vi "Frames.vi"(8 "error in (no error)":errorcluster, 11 "Node Ptr":T1 format="%.0x") -> (0 "error out":errorcluster)   [LabVIEW 2019, in "Diagnostics Addon System Explorer.lvlib"]
uses:
  Diagnostics Addon System Explorer.lvlib
  <vilib>/NI VeriStand/Custom Device API/Custom Device Item Ref.ctl
  Types/FG.Action.ctl
  Addon Shared/SubVIs/Constants.vi
  <vilib>/NI/NI VeriStand Advanced SysDef API/SysDef API/SysDef.Property.Set.vi
  <vilib>/NI/NI VeriStand Advanced SysDef API/_SubVIs/SysDef.Property.Set.U32.vi
  <vilib>/NI VeriStand/Custom Device API/NI VeriStand - Get Item Property.vi
  <vilib>/NI VeriStand/Custom Device API/Get Item Property (U32).vi
  <vilib>/NI VeriStand/Custom Device API/Custom Device API.lvlib
  Addon Shared/Diagnostics Addon Shared.lvlib
panel:
  in  "Description":string
  in  "SHDocVw.IWebBrowser":refnum<k7>(container)
  out "Frames":i32(listbox)
  out "Name":string
  in  "Header":cluster{"Section Name":string}={"Section Name"="Custom Device Item Settings"}
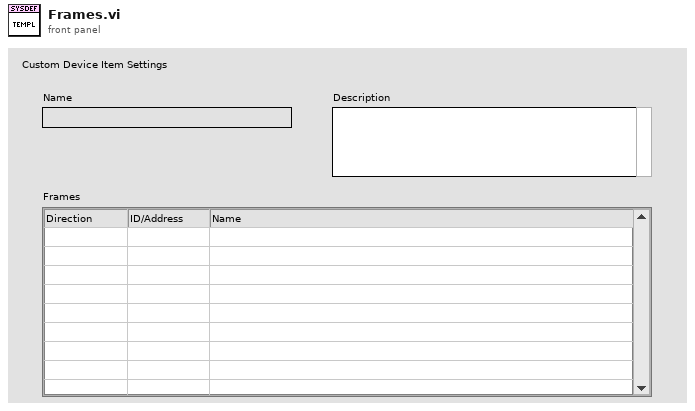
[diagram p1: front panel]
types:
  T1 = typedef "Custom Device API.lvlib/Custom Device Item Ref.ctl" = u64
  T2 = typedef "Diagnostics Addon System Explorer.lvlib/FG.Action.ctl" = enum16{"Get", "Set"}
  T3 = typedef "Custom Device API.lvlib/Custom Device Item Info.ctl" = cluster{"Name":string, "Is Channel":bool, "GUID":string, "Is Waveform":bool}
  T4 = typedef "Custom Device API.lvlib/Custom Device Commands.ctl" = enum16{"Default", "Item renamed", "Shutdown", "Dynamic button pressed"}
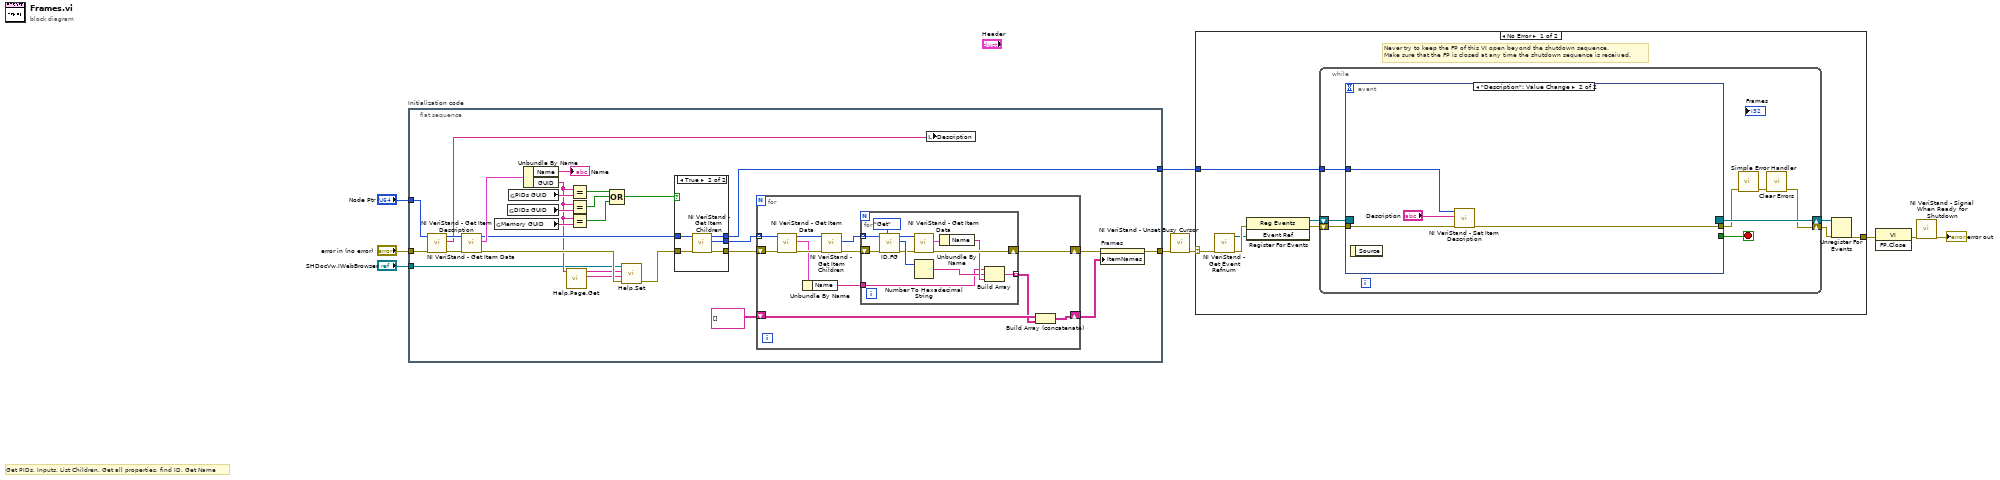
[diagram p0: block diagram]
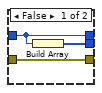
[diagram p2: hidden frame]
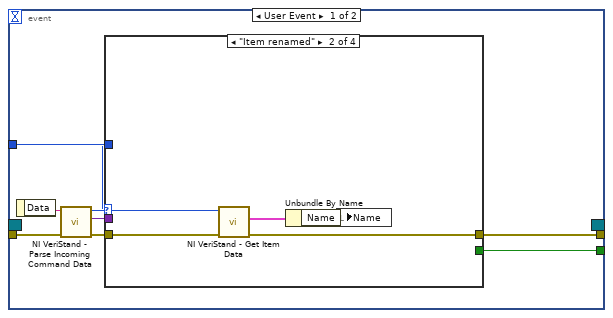
[diagram p3: hidden frame]
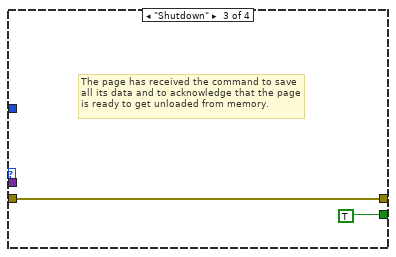
[diagram p5: hidden frame]
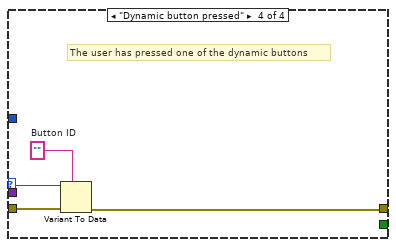
[diagram p6: hidden frame]
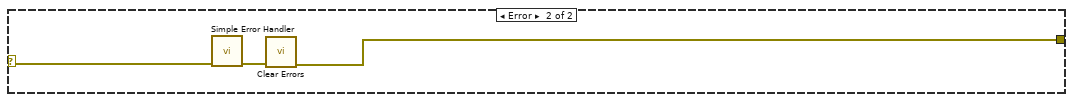
[diagram p7: hidden frame]
diagram:
  # "Get PIDs, Inputs, List Children, Get all properties, find ID, Get Name"
  n1 = flat-sequence "Initialization code" {
    tunnel: "error in (no error)" -> [w23]
    tunnel: "Node Ptr" -> [w36]
    tunnel: [w32] -> w5
    tunnel: [w29] -> w2
    tunnel: "SHDocVw.IWebBrowser" -> [w11]
    frame #0 {
      n2 = call <vilib>:"NI VeriStand - Get Item Description.vi"("error in (no error)"=w23, "Item Ref in"=w36) -> ("error out"=w35:errorcluster, "Description"=w24:string, "Item Ref out"=w37:T1)  [unwired: 7 out]
      n3 = call <vilib>:"NI VeriStand - Get Item Data.vi"("error in (no error)"=w35, "Item Ref in"=w37) -> ("error out"=w22:errorcluster, "Item Info"=w34:T3, "Item Ref out"=w31:T1)  [unwired: 7 out]
      n4 = global read "Constants.vi" "Memory GUID"() -> (w18:string)
      n5 = global read "Constants.vi" "DIDs GUID"() -> (w16:string)
      n6 = global read "Constants.vi" "PIDs GUID"() -> (w15:string)
      n7 = Unbundle By Name(w34) -> ("Name"=→"Name":string, "GUID"=w13:string)
      n8 = call "Help.Page.Get.vi"("GUID"=w13) -> ("HTML File"=w12:string, "Main CHM File"=w10:string)  [unwired: 9 in]
      n9 = Equal?(x=w13, y=w15) -> (x = y?=w20:bool)
      n10 = Equal?(x=w13, y=w16) -> (x = y?=w17:bool)
      n11 = Equal?(x=w13, y=w18) -> (x = y?=w19:bool)
      n12 = Compound Arithmetic op=OR(w20, w17, w19) -> (w14:bool)
      n13 = call "Help.Set.vi"("error in (no error)"=w22, "HTML File"=w12, "Main CHM File"=w10, "SHDocVw.IWebBrowser2"=w11) -> ("error out"=w21:errorcluster)  [unwired: 7 in]
      n14 = case shown="True" w14 {
        tunnel: w21 -> [w40 w45]
        tunnel: w31 -> [w39 w44]
        tunnel: [w40 w43] -> w30
        tunnel: [w39 w42] -> w29
        tunnel: [w38 w41] -> w28
        frame False {
          n15 = Build Array(w39) -> (w38:T1[])
        }
        frame True {
          n16 = call <vilib>:"NI VeriStand - Get Item Children.vi"("error in (no error)"=w45, "Item Ref in"=w44) -> ("error out"=w43:errorcluster, "Child Refs"=w41:T1[], "Item Ref out"=w42:T1)  [unwired: 6 in, 1 out]
        }
      }
      n17 = for {
        tunnel: w28 -> [w49] mode=indexing
        shift-right: [w57] -> w33
        shift-left: w30 -> [w54]
        shift-right: [w46] -> w26
        shift-left: string[][] [] -> [w48]
        n18 = call <vilib>:"NI VeriStand - Get Item Data.vi"("error in (no error)"=w54, "Item Ref in"=w49) -> ("error out"=w53:errorcluster, "Item Info"=w51:T3, "Item Ref out"=w52:T1)  [unwired: 7 out]
        n19 = Unbundle By Name(w51) -> ("Name"=w50:string)
        n20 = call <vilib>:"NI VeriStand - Get Item Children.vi"("error in (no error)"=w53, "Item Ref in"=w52) -> ("error out"=w55:errorcluster, "Child Refs"=w56:T1[])  [unwired: 6 in, 2 out]
        n21 = for {
          tunnel: w56 -> [w69] mode=indexing
          shift-right: [w65] -> w57
          shift-left: w55 -> [w68]
          tunnel: [w60] -> w47 mode=indexing
          tunnel: w50 -> [w59]
          n22 = call "ID.FG.vi"("Action"=FG.Action."Get", "error in (no error)"=w68, "Device Item Ref in"=w69) -> ("error out"=w66:errorcluster, "ID"=w67:u32, "Device Item Ref out"=w64:T1)  [unwired: 6 in]
          n23 = call <vilib>:"NI VeriStand - Get Item Data.vi"("error in (no error)"=w66, "Item Ref in"=w64) -> ("error out"=w65:errorcluster, "Item Info"=w63:T3)  [unwired: 8 out]
          n24 = Number To Hexadecimal String(2:w67) -> (0:w61:string)  [unwired: 1 in]
          n25 = Unbundle By Name(w63) -> ("Name"=w62:string)
          n26 = Build Array(w59, w61, w62) -> (w60:string[])
        }
        n27 = Build Array (concatenate)(w48, w47) -> (w46:string[][])
      }
      n28 = local write "Description"(w24) -> ()
      n29 = property on="Frames" class="MCListbox (strict)"(error in=w33, "ItemNames"=w26) -> (error out=w32:errorcluster)  [unwired: 1 in, 1 out]
    }
  }
  n30 = call <vilib>:"NI VeriStand - Unset Busy Cursor.vi"("error in (no error)"=w5) -> ("error out"=w4:errorcluster)  [unwired: 10 out]
  n31 = case shown="No Error" w4 {
    selector: w4 -> [w70 w113]
    tunnel: [w75 w111] -> w9
    tunnel: w2 -> [w71 _]
    frame No Error {
      # "Never try to keep the FP of this VI open beyond the shutdown sequence.\nMake sure that the FP is closed at any time the shutdown sequence is received."
      n32 = call <vilib>:"NI VeriStand - Get Event Refnum.vi"("error in (no error)"=w70) -> ("error out"=w78:errorcluster, "Event Ref"=w74:refnum<user-event>)  [unwired: 9 out]
      n33 = register-events(error in=w78, w74) -> (reference out=w72:refnum<event-registration>, error out=w73:errorcluster)  [unwired: 1 in]
      n34 = while {
        tunnel: w71 -> [w82]
        shift-right: [w79] -> w76
        shift-left: w73 -> [w85]
        shift-right: [w86] -> w77
        shift-left: w72 -> [w84]
        stop <- w83 stop-if-true
        n35 = event shown="[1] \"Description\": Value Change" {
          selector: w84 -> [_ _]
          dyn-events: [_ _] -> w86
          timeout: _ -> [_ _]
          tunnel: w85 -> [w94 w109]
          tunnel: [w90 _] -> w83
          tunnel: [w89 w107] -> w81
          tunnel: w82 -> [w88 w110]
          event User Event {
            n36 = event-data() -> ("Data"=w93:string)  [unwired: 1 out]
            n37 = call <vilib>:"NI VeriStand - Parse Incoming Command Data.vi"("error in (no error)"=w94, "Incoming data"=w93) -> ("error out"=w92:errorcluster, "Outgoing data"=w87:variant, "Action"=w91:T4)  [unwired: 7 out]
            n38 = case shown="\"Item renamed\"" w91 {
              tunnel: w92 -> [w95 w100 w101 w106]
              tunnel: [_ _ TRUE _] -> w90
              tunnel: [w95 w97 w101 w103] -> w89
              tunnel: w88 -> [_ w99 _ _]
              tunnel: w87 -> [_ _ _ w105]
              frame "Default", Default {
              }
              frame "Item renamed" {
                n39 = call <vilib>:"NI VeriStand - Get Item Data.vi"("error in (no error)"=w100, "Item Ref in"=w99) -> ("error out"=w97:errorcluster, "Item Info"=w98:T3)  [unwired: 8 out]
                n40 = Unbundle By Name(w98) -> ("Name"=w96:string)
                n41 = local write "Name"(w96) -> ()
              }
              frame "Shutdown" {
                # "The page has received the command to save all its data and to acknowledge that the page is ready to get unloaded from memory."
              }
              frame "Dynamic button pressed" {
                w104 = ""  # Button ID
                # "The user has pressed one of the dynamic buttons"
                n42 = Variant To Data(error in=w106, type=w104, Variant=w105) -> (error out=w103:errorcluster)  [unwired: 1 out]
              }
            }
          }
          event "Description": Value Change {
            n43 = event-data() -> ()  [unwired: 2 out]
            n44 = call <vilib>:"NI VeriStand - Set Item Description.vi"("error in (no error)"=w109, "Description"="Description", "Item Ref in"=w110) -> ("error out"=w107:errorcluster)  [unwired: 8 out]
          }
        }
        n45 = call <vilib>:"Simple Error Handler.vi"("error in (no error)"=w81) -> ("error out"=w80:errorcluster)  [unwired: 1 in, 7 out]
        n46 = call <vilib>:"Clear Errors.vi"("error in (no error)"=w80) -> ("error out"=w79:errorcluster)  [unwired: 1 in, 5 out]
      }
      n47 = Unregister For Events(event registration refnum=w77, error in=w76) -> (error out=w75:errorcluster)
    }
    frame Error {
      n48 = call <vilib>:"Simple Error Handler.vi"("error in (no error)"=w113) -> ("error out"=w112:errorcluster)  [unwired: 1 in, 7 out]
      n49 = call <vilib>:"Clear Errors.vi"("error in (no error)"=w112) -> ("error out"=w111:errorcluster)  [unwired: 1 in, 5 out]
    }
  }
  n50 = invoke class="VI" method="FP.Close"(error in=w9) -> (error out=w8:errorcluster)  [unwired: 2 in, 2 out]
  n51 = call <vilib>:"NI VeriStand - Signal When Ready for Shutdown.vi"("error in (no error)"=w8) -> ("error out"=→"error out":errorcluster)  [unwired: 10 out]
